vi "属性节点（波形图表）.vi"() -> ()   [LabVIEW 2017]
panel:
  in  "停止":bool
  out "波形图表":dbl(graph)
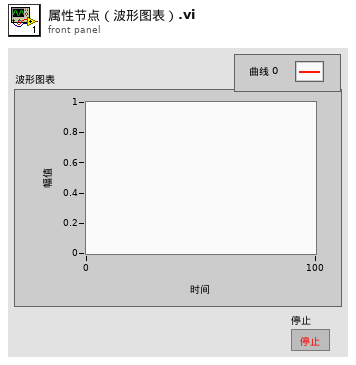
[diagram p1: front panel]
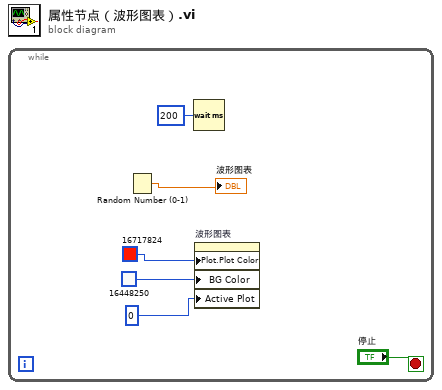
[diagram p0: block diagram]
diagram:
  n1 = while {
    stop <- "停止" stop-if-true
    n2 = Random Number (0-1)() -> (number: 0 to 1=→"波形图表":dbl)
    n3 = Wait (ms)(milliseconds to wait=u32 200 ("等待时间（毫秒）")) -> ()  [unwired: 1 out]
    n4 = property on="波形图表" class="WFChart (严格)"("Plot.Plot Color"=u32 16717824, "BG Color"=u32 16448250, "Active Plot"=0) -> ()  [unwired: 2 in, 2 out]
  }
